vi "test2.vi"   [LabVIEW 2020]
uses:
  14239ad6-c32a-4ff8-8a04-f737b7f50bb8.vi
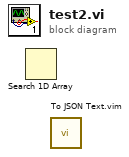
[diagram p0: block diagram]
diagram:
  n1 = Search 1D Array ("搜索一维数组")() -> ()  [unwired: 3 in, 1 out]
  n2 = call "To JSON Text.vim"() -> ()  [unwired: 10 in, 2 out]
